vi "abre pdf - exemplo.vi"() -> ()   [LabVIEW 2019]
panel:
  out "string":string
  out "LoadFile":bool
  in  "path":path
  in  "AcroPDF":refnum<k7>(container)
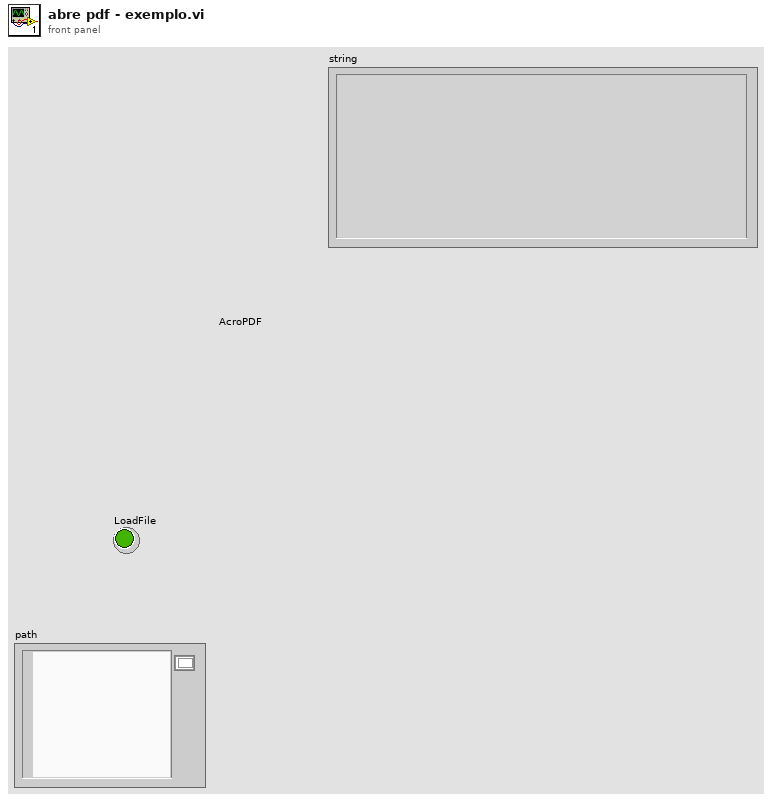
[diagram p1: front panel]
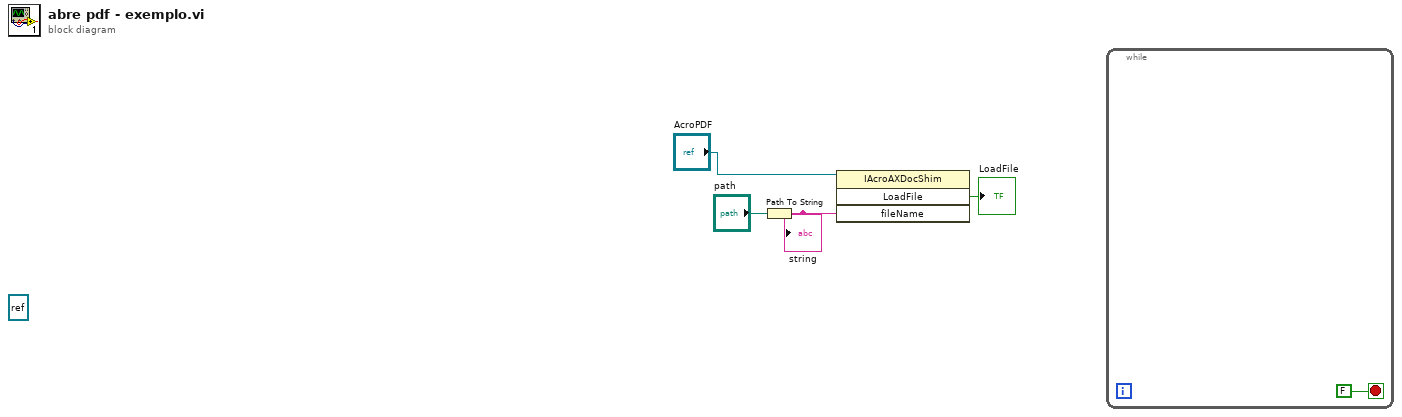
[diagram p0: block diagram]
diagram:
  (unwired) refnum<k7> refnum ("AcroPDF")
  n1 = Path To String(path="path") -> (string=w3:string)
  "string" <- w3
  n2 = invoke class="IAcroAXDocShim" method="LoadFile"(reference="AcroPDF", "fileName"=w3) -> ("LoadFile"=→"LoadFile":bool)  [unwired: 2 in, 3 out]
  n3 = while {
    stop <- FALSE stop-if-true
  }
